vi "NewTableBuild.vi"() -> ()   [LabVIEW 2012]
uses:
  Controls/WaferTable.ctl
  Controls/Measurement.ctl
  Controls/TestData.ctl
panel:
  out "input cluster":T1 {"50mA Data"."Reverse" format="%#_3g"; "50mA Data"."Current,mA" format="%_6g"; "50mA Data"."Knee Current" format="%#_3g"; "50mA Data"."WL" format="%_6g"; "50mA Data"."Voltage" format="%_6g"; "50mA Data"."Power" format="%_5g"; "20mA Data"."Reverse" format="%#_3g"; "20mA Data"."Current,mA" format="%_6g"; "20mA Data"."Knee Current" format="%#_3g"; "20mA Data"."WL" format="%_6g"; "20mA Data"."Voltage" format="%_6g"; "20mA Data"."Power" format="%_5g"}
  out "20mA Data":T2 {"Reverse" format="%#_3g"; "Current,mA" format="%_6g"; "Knee Current" format="%#_3g"; "WL" format="%_6g"; "Voltage" format="%_6g"; "Power" format="%_5g"}
  in  "WaferTable":T3
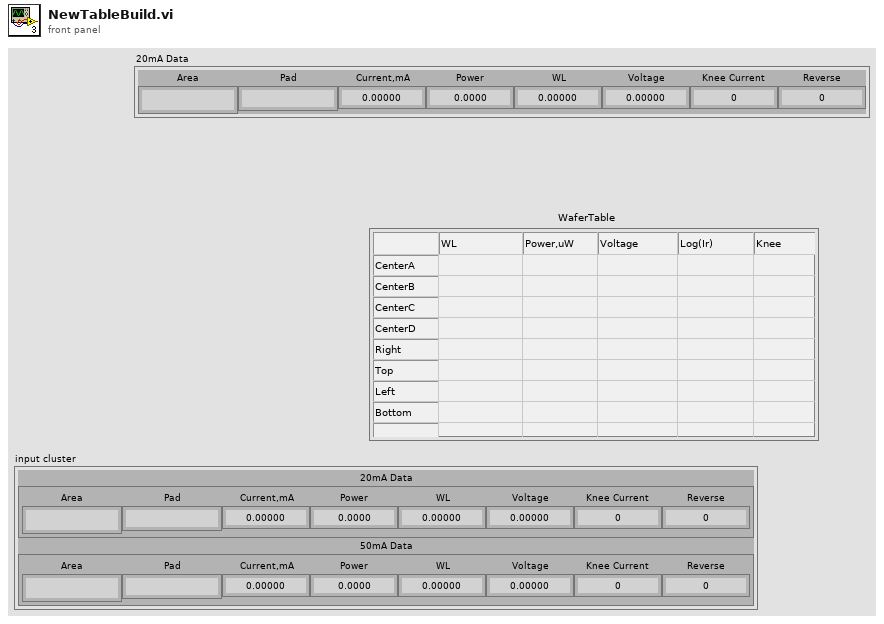
[diagram p1: front panel]
types:
  T1 = typedef "TestData.ctl" = cluster{"20mA Data":T2, "50mA Data ":T2}
  T2 = typedef "Measurement.ctl" = cluster{"Area":string, "Pad":string, "Current,mA":dbl, "Power":dbl, "WL":dbl, "Voltage":dbl, "Knee Current":dbl, "Reverse":dbl}
  T3 = typedef "WaferTable.ctl" = string[][]
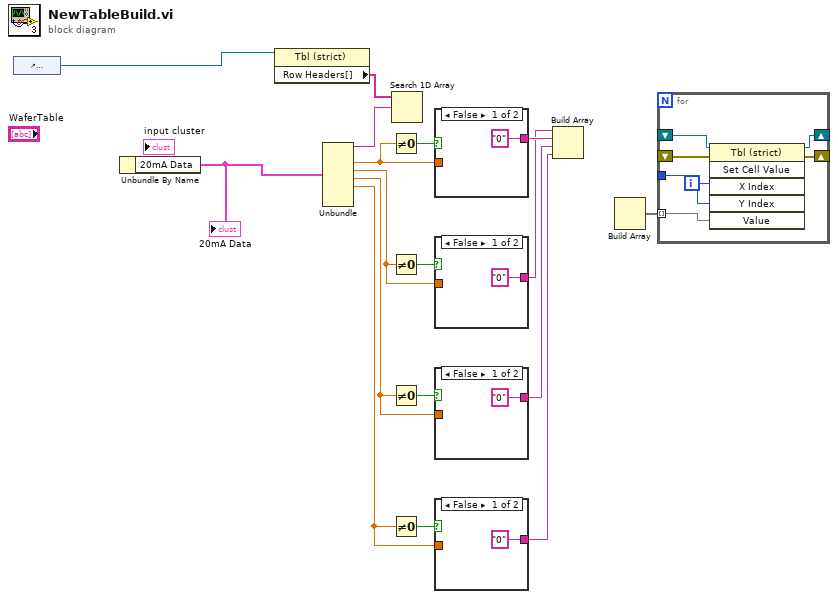
[diagram p0: block diagram]
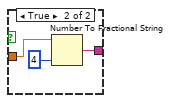
[diagram p2: hidden frame]
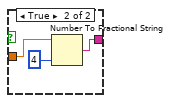
[diagram p3: hidden frame]
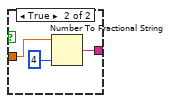
[diagram p4: hidden frame]
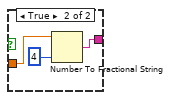
[diagram p5: hidden frame]
diagram:
  n1 = control-ref of="WaferTable"() -> (w2:refnum<vi>)
  n2 = Unbundle By Name() -> ("20mA Data"=w17:T2)  [unwired: 1 in]
  "20mA Data" <- w17
  n3 = property class="Tbl (strict)"(reference=w2) -> ("Row Headers[]"=w16:string[])  [unwired: 1 in, 2 out]
  n4 = Unbundle(w17) -> ("Area"=w15:string, "Current,mA"=w13:dbl, "Power"=w7:dbl, "WL"=w8:dbl, "Voltage"=w9:dbl)  [unwired: 3 out]
  n5 = Not Equal To 0?(x=w13) -> (x != 0?=w14:bool)
  n6 = Not Equal To 0?(x=w7) -> (x != 0?=w12:bool)
  n7 = Not Equal To 0?(x=w8) -> (x != 0?=w11:bool)
  n8 = Not Equal To 0?(x=w9) -> (x != 0?=w10:bool)
  n9 = Search 1D Array(1D array=w16, element=w15) -> ()  [unwired: 1 in, 1 out]
  n10 = case shown="False" w14 {
    tunnel: w13 -> [_ w21]
    tunnel: ["0" ("F-format string") w19] -> w6
    frame False {
    }
    frame True {
      n11 = Number To Fractional String(number=w21, precision (6)=i16 4) -> (F-format string=w19:string)  [unwired: 2 in]
    }
  }
  n12 = case shown="False" w12 {
    tunnel: ["0" ("F-format string") w24] -> w5
    tunnel: w7 -> [_ w23]
    frame False {
    }
    frame True {
      n13 = Number To Fractional String(number=w23, precision (6)=i16 4) -> (F-format string=w24:string)  [unwired: 2 in]
    }
  }
  n14 = case shown="False" w11 {
    tunnel: ["0" ("F-format string") w28] -> w4
    tunnel: w8 -> [_ w27]
    frame False {
    }
    frame True {
      n15 = Number To Fractional String(number=w27, precision (6)=i16 4) -> (F-format string=w28:string)  [unwired: 2 in]
    }
  }
  n16 = case shown="False" w10 {
    tunnel: ["0" ("F-format string") w32] -> w3
    tunnel: w9 -> [_ w31]
    frame False {
    }
    frame True {
      n17 = Number To Fractional String(number=w31, precision (6)=i16 4) -> (F-format string=w32:string)  [unwired: 2 in]
    }
  }
  n18 = Build Array(w5, w6, w4, w3) -> ()  [unwired: 1 out]
  n19 = Build Array() -> (w1:void[])  [unwired: 4 in]
  n20 = for {
    tunnel: w1 -> [w37] mode=indexing
    tunnel: _ -> [w39]
    shift-right: [w35] -> _
    shift-left: _ -> [w36]
    shift-right: [w34] -> _
    shift-left: _ -> [w40]
    i -> [w38]
    n21 = invoke class="Tbl (strict)" method="Set Cell Value"(reference=w40, error in=w36, "X Index"=w38, "Y Index"=w39, "Value"=w37) -> (reference out=w34:refnum<vi>, error out=w35:errorcluster)  [unwired: 1 in, 4 out]
  }
